vi "resistance-global.vi"() -> ()   [LabVIEW 2013]
panel:
  in  "Resistance Array":dbl[](array[numeric])
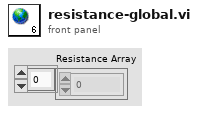
[diagram p1: front panel]
diagram:
